vi "Edit Instructions File.vi"(0 "Instruction File Path":path=path "D:/modernlab-ref-architecture/src/measurement_build_automation/_Measurement Builder/Template for Package/data/instructions", 5 "Measurement Name":string, 11 "error in (no error)":errorcluster) -> (15 "error out":errorcluster)   [LabVIEW 2021, in "Packager Helpers.lvlib"]
uses:
  Packager Helpers.lvlib
  <vilib>/Utility/sysdir.llb/System Directory Type.ctl
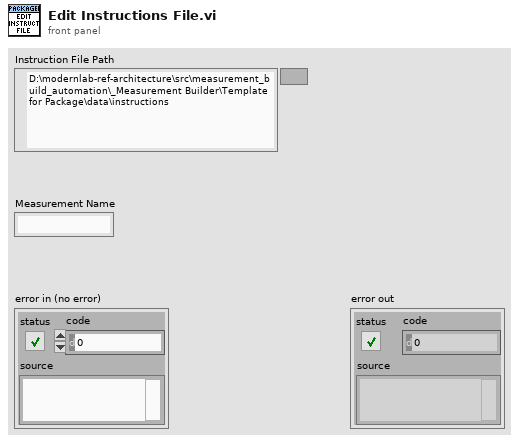
[diagram p1: front panel]
types:
  T1 = enum16{"open", "replace", "create", "open or create", "replace or create", "replace or create with confirmation"}
  T2 = typedef "System Directory Type.ctl" = i32
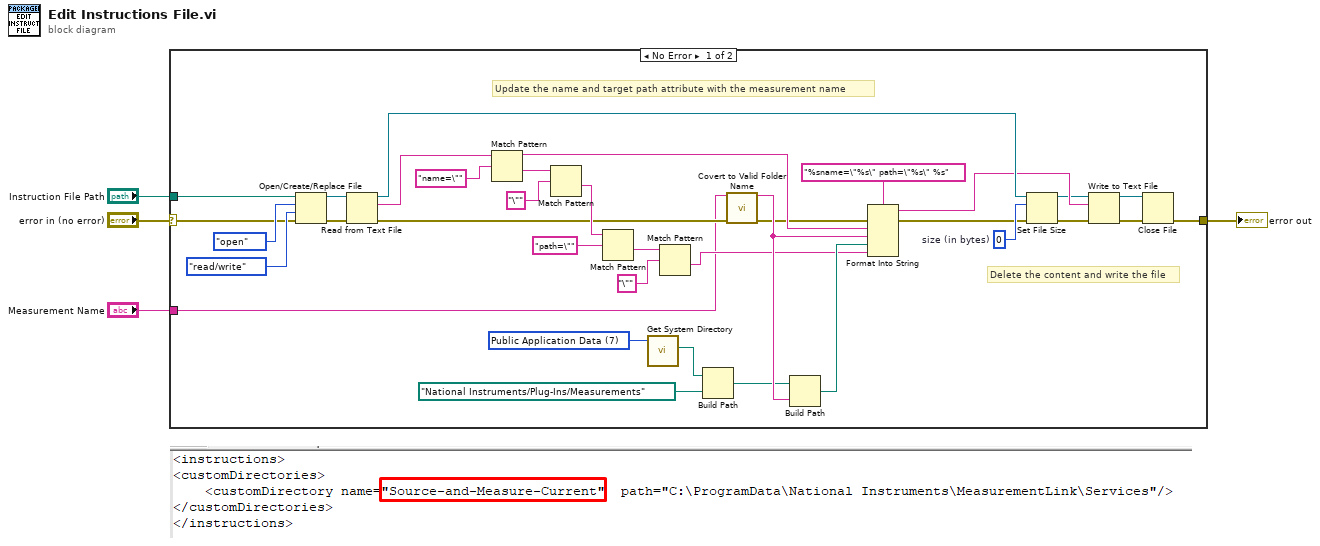
[diagram p0: block diagram]
diagram:
  n1 = case shown="No Error" "error in (no error)" {
    selector: "error in (no error)" -> [w18 w40]
    tunnel: "Instruction File Path" -> [w39 _]
    tunnel: [w5 w40] -> w1
    tunnel: "Measurement Name" -> [w7 _]
    frame No Error {
      w19 = T2 7 items=["User Home"=0, "User Desktop"=1, "User Documents"=2, "User Application Data"=3, "User Preferences"=4, "User Temporary"=5, "Public Documents"=6, "Public Application Data"=7, "Public Preferences"=8, "Public Cache"=13, "System Core Libraries"=9, "System Installed Libraries"=10, "Application Files"=11, "Boot Volume Root"=12] ("system directory type")
      w28 = i64 0  # size (in bytes)
      # "Delete the content and write the file"
      # "Update the name and target path attribute with the measurement name"
      n2 = Open/Create/Replace File(file path (use dialog)=w39, error in=w18, operation (0:open)=T1."open", access (0:read/write)=enum16{"read/write", "read-only", "write-only"}."read/write") -> (refnum out=w36:refnum<file>, error out=w17:errorcluster)  [unwired: 2 in, 1 out]
      n3 = Read from Text File(file (use dialog)=w36, error in=w17) -> (refnum out=w29:refnum<file>, text=w35:string, error out=w16:errorcluster)  [unwired: 2 in, 1 out]
      n4 = Match Pattern(string=w35, regular expression="name=\"") -> (before substring=w30:string, after substring=w33:string)  [unwired: 1 in, 2 out]
      n5 = Match Pattern(string=w33, regular expression="\"") -> (after substring=w27:string)  [unwired: 1 in, 3 out]
      n6 = Match Pattern(string=w27, regular expression="path=\"") -> (after substring=w9:string)  [unwired: 1 in, 3 out]
      n7 = call <vilib>:"Get System Directory.vi"("system directory type"=w19) -> ("system directory"=w22:path)  [unwired: 10 in]
      n8 = Match Pattern(string=w9, regular expression="\"") -> (after substring=w23:string)  [unwired: 1 in, 3 out]
      n9 = Build Path(base path=w22, name or relative path=path "National Instruments/Plug-Ins/Measurements" ("Instruction File")) -> (appended path=w21:path)
      n10 = call "Covert to Valid Folder Name.vi"("Folder Name"=w7, "error in (no error)"=w16) -> ("Valid Folder Name"=w25:string, "error out"=w15:errorcluster)  [unwired: 12 in]
      n11 = Build Path(base path=w21, name or relative path=w25) -> (appended path=w24:path)
      n12 = Format Into String(format string="%sname=\"%s\" path=\"%s\" %s", error in=w15, w30, w25, w24, w23) -> (resulting string=w12:string, error out=w14:errorcluster)  [unwired: 1 in]
      n13 = Set File Size(4:w14, 6:w28, 7:w29) -> (0:w13:errorcluster, 3:w11:refnum<file>)
      n14 = Write to Text File(file (use dialog)=w11, text=w12, error in=w13) -> (refnum out=w10:refnum<file>, error out=w6:errorcluster)  [unwired: 1 in, 1 out]
      n15 = Close File(refnum=w10, error in=w6) -> (error out=w5:errorcluster)  [unwired: 1 out]
    }
    frame Error {
    }
  }
  "error out" <- w1
